vi "GetChannelName.vi"(8 "error in (no error)":errorcluster, 11 "ClassIn":refnum<class "NiPxi6733.lvclass">) -> (0 "error out":errorcluster, 3 "ClassOut":refnum<class "NiPxi6733.lvclass">)   [LabVIEW 2014, in "FGenPlugins.lvlib" / "NiPxi6733.lvclass"]
uses:
  NiPxi6733.lvclass
  MyPluginBaseClass/TypeDef/ChannelParamElement.ctl
  <vilib>/Utility/error.llb/Error Cluster From Error Code.vi
  <vilib>/ErrorRing/Error Ring.xnode
  MyPluginBaseClass/NISTFGenPluginsBase.lvclass
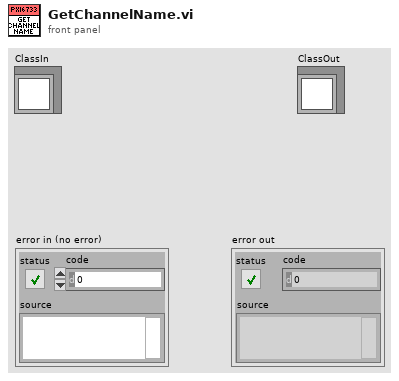
[diagram p1: front panel]
types:
  T1 = typedef "FGenPlugins.lvlib/NISTFGenPluginsBase.lvclass/ChannelParamElement.ctl" = cluster{"sName":string, "eOperateMode":u16, "bEnabled":bool, "eOutputMode":u16, "iIndex":i32, "iNameBufferSize":i32, "fGain":dbl}
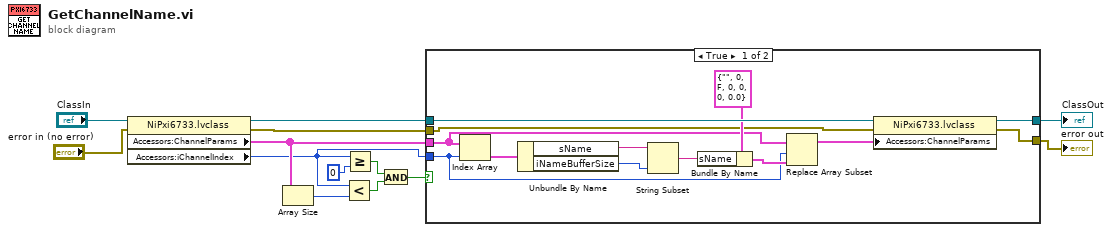
[diagram p0: block diagram]
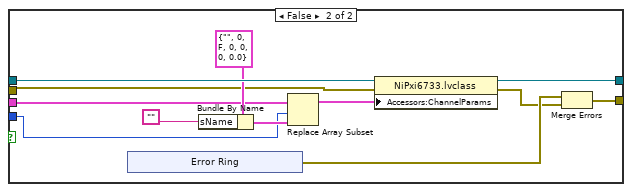
[diagram p2: hidden frame]
diagram:
  n1 = property class="NiPxi6733.lvclass"(reference="ClassIn", error in="error in (no error)") -> (reference out=w7:refnum<class "NiPxi6733.lvclass">, error out=w6:errorcluster, "Accessors:ChannelParams"=w12:T1[], "Accessors:iChannelIndex"=w5:i32)
  n2 = Array Size(array=w12) -> (size(s)=w11:i32)
  n3 = Less?(x=w5, y=w11) -> (x < y?=w10:bool)
  n4 = Greater Or Equal?(x=w5, y=0 ("x")) -> (x >= y?=w13:bool)
  n5 = And(x=w13, y=w10) -> (x .and. y?=w9:bool)
  n6 = case shown="True" w9 {
    tunnel: w12 -> [w19 w35]
    tunnel: w7 -> [w23 w38]
    tunnel: [w17 w33] -> w2
    tunnel: w6 -> [w16 w32]
    tunnel: [w15 w27] -> w1
    tunnel: w5 -> [w14 w30]
    frame True {
      n7 = Index Array(array=w19, index=w14) -> (element=w26:T1)
      n8 = Unbundle By Name(w26) -> ("sName"=w25:string, "iNameBufferSize"=w24:i32)
      n9 = String Subset(string=w25, length (rest)=w24) -> (substring=w22:string)  [unwired: 1 in]
      n10 = Bundle By Name(cluster=T1 {"sName"="", "eOperateMode"=0, "bEnabled"=FALSE, "eOutputMode"=0, "iIndex"=0, "iNameBufferSize"=0, "fGain"=0.0} ("ChannelParamElement"), "sName"=w22) -> (w20:T1)
      n11 = Replace Array Subset(array=w19, new element=w20, index=w14) -> (w18:T1[])
      n12 = property class="NiPxi6733.lvclass"(reference=w23, error in=w16, "Accessors:ChannelParams"=w18) -> (reference out=w17:refnum<class "NiPxi6733.lvclass">, error out=w15:errorcluster)
    }
    frame False {
      n13 = xnode "Error Ring"() -> ("error out"=w29:errorcluster)
      n14 = Bundle By Name(cluster=T1 {"sName"="", "eOperateMode"=0, "bEnabled"=FALSE, "eOutputMode"=0, "iIndex"=0, "iNameBufferSize"=0, "fGain"=0.0} ("ChannelParamElement"), "sName"="") -> (w36:T1)
      n15 = Replace Array Subset(array=w35, new element=w36, index=w30) -> (w34:T1[])
      n16 = property class="NiPxi6733.lvclass"(reference=w38, error in=w32, "Accessors:ChannelParams"=w34) -> (reference out=w33:refnum<class "NiPxi6733.lvclass">, error out=w28:errorcluster)
      n17 = Merge Errors(w29, w28) -> (w27:errorcluster)
    }
  }
  "error out" <- w1
  "ClassOut" <- w2
